vi "LEP_RV_ExtInt_Config.vi"(8 "error in (no error)":errorcluster, 10 "configuration":string[](array[string]), 11 "interrupt name":string) -> (0 "error out":errorcluster, 3 "configuration":string[](array[string]))   [LabVIEW 2011]
panel:
  in  "help":bool
  in  "cancel":bool
  in  "ok":bool
  in  "Interrupt Type":T1(ring)
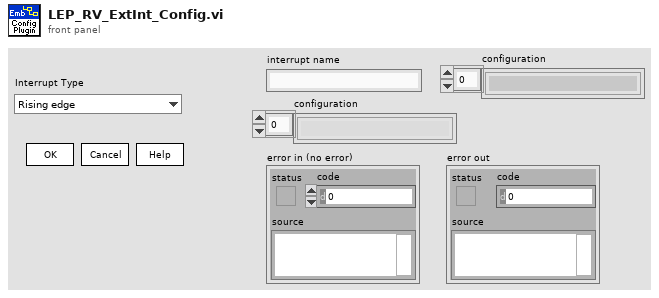
[diagram p1: front panel]
types:
  T1 = enum16{"Rising edge", "Falling edge", "High level", "Low level"}
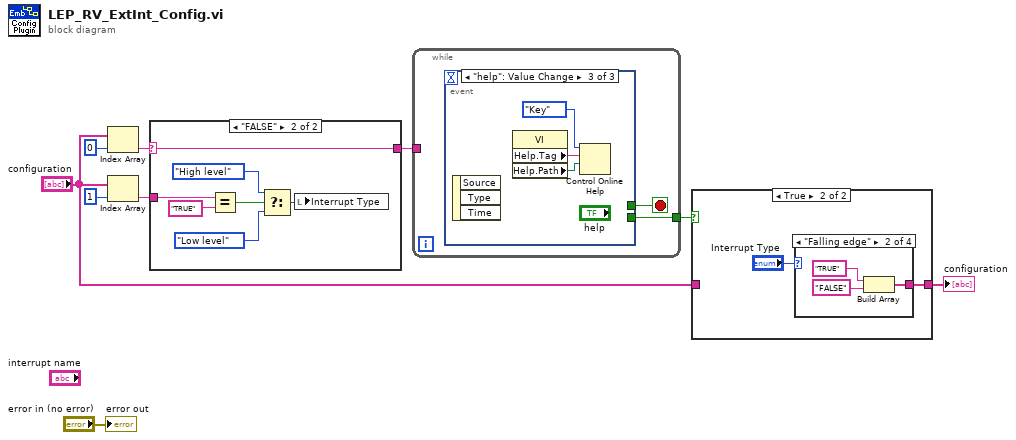
[diagram p0: block diagram]
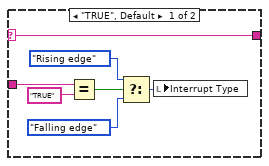
[diagram p2: hidden frame]
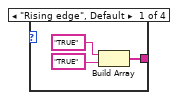
[diagram p4: hidden frame]
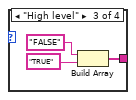
[diagram p5: hidden frame]
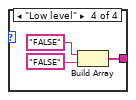
[diagram p6: hidden frame]
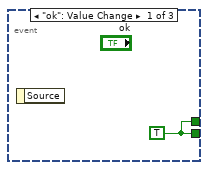
[diagram p7: hidden frame]
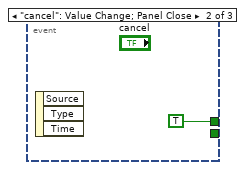
[diagram p8: hidden frame]
diagram:
  n1 = Index Array(array="configuration", index=0) -> (element=w3:string)
  n2 = Index Array(array="configuration", index=1) -> (element=w2:string)
  n3 = case shown="\"FALSE\"" w3 {
    selector: w3 -> [w13 w20]
    tunnel: w2 -> [w15 w22]
    tunnel: [w13 w20] -> w1
    frame "TRUE", Default {
      n4 = Equal?(x=w15, y="TRUE") -> (x = y?=w14:bool)
      n5 = Select(t=T1."Rising edge" ("Interrupt Type"), s=w14, f=T1."Falling edge" ("Interrupt Type")) -> (s? t:f=w10:T1)
      n6 = local write "Interrupt Type"(w10) -> ()
    }
    frame "FALSE" {
      n7 = Equal?(x=w22, y="TRUE") -> (x = y?=w21:bool)
      n8 = Select(t=T1."High level" ("Interrupt Type"), s=w21, f=T1."Low level" ("Interrupt Type")) -> (s? t:f=w17:T1)
      n9 = local write "Interrupt Type"(w17) -> ()
    }
  }
  n10 = while {
    tunnel: [w24] -> w8
    tunnel: w1 -> [_]
    stop <- w25 stop-if-true
    n11 = event shown="[2] \"help\": Value Change" {
      selector: _ -> [_ _ _]
      dyn-events: _ -> [_ _ _]
      timeout: _ -> [_ _ _]
      tunnel: [w26 TRUE _] -> w25
      tunnel: [w26 _ _] -> w24
      event "ok": Value Change {
        w26 = TRUE
        n12 = event-data() -> ()  [unwired: 2 out]
      }
      event "cancel": Value Change; Panel Close {
        n13 = event-data() -> ()  [unwired: 4 out]
      }
      event "help": Value Change {
        n14 = event-data() -> ()  [unwired: 4 out]
        n15 = property class="VI"() -> ("Help.Tag"=w28:string, "Help.Path"=w29:path)  [unwired: 2 in, 2 out]
        n16 = Control Online Help(2:w29, 3:w28, 4:enum16{"Contents", "Key", "Close"}."Key" ("Operation")) -> ()  [unwired: 1 in, 1 out]
      }
    }
  }
  n17 = case shown="True" w8 {
    tunnel: [w31 w32] -> w7
    tunnel: "configuration" -> [w31 _]
    frame False {
    }
    frame True {
      n18 = case shown="\"Falling edge\"" "Interrupt Type" {
        tunnel: [w34 w37 w40 w43] -> w32
        frame "Rising edge", Default {
          n19 = Build Array("TRUE", "TRUE") -> (w34:string[])
        }
        frame "Falling edge" {
          n20 = Build Array("TRUE", "FALSE") -> (w37:string[])
        }
        frame "High level" {
          n21 = Build Array("FALSE", "TRUE") -> (w40:string[])
        }
        frame "Low level" {
          n22 = Build Array("FALSE", "FALSE") -> (w43:string[])
        }
      }
    }
  }
  "configuration" <- w7
  "error out" <- "error in (no error)"
